vi "ztscopeM Read Waveform Preamble.vi"(0 "Instrument Handle In":i32, 5 "Source":i32(ring) items=["Input Channel 1", "Input Channel 2", "Input Channel 3", "Input Channel 4", "Calc Channel 1", "Calc Channel 2", "Calc Channel 3", "Calc Channel 4", "Ref Channel 1", "Ref Channel 2", "Ref Channel 3", "Ref Channel 4"], 11 "error in":errorcluster) -> (2 "Voltage Offset":dbl, 3 "Voltage Interval":dbl, 4 "Instrument Handle Out":i32, 6 "Type":i32=1, 8 "Points":u32=100, 10 "Acquisition Count":i32=1, 13 "Time Offset":dbl, 14 "Time Interval":dbl=9.99999993922529e-09, 15 "error out":errorcluster)   [LabVIEW 2013]
doc: "Query the selected channel's preamble. The preamble contains all the information necessary to retrieve and interpret a waveform readback."
uses:
  ztscopeM.dll
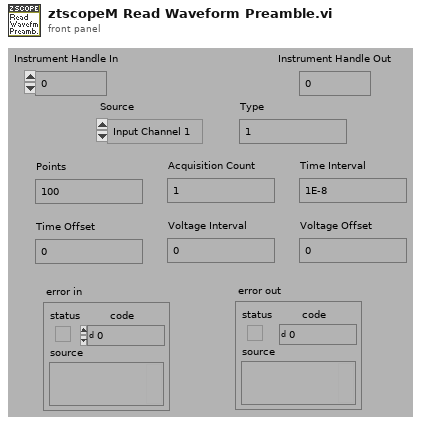
[diagram p1: front panel]
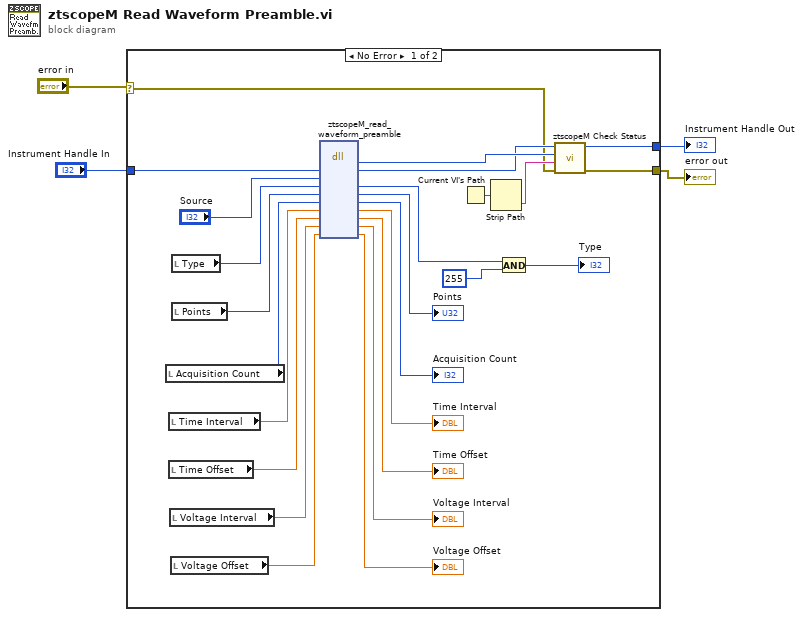
[diagram p0: block diagram]
diagram:
  n1 = case shown="No Error" "error in" {
    selector: "error in" -> [w12 w31]
    tunnel: [w11 w31] -> w1
    tunnel: "Instrument Handle In" -> [w29 w30]
    tunnel: [w10 w30] -> w3
    frame No Error {
      n2 = local read "Acquisition Count"() -> (w24:i32)
      n3 = local read "Time Interval"() -> (w22:dbl)
      n4 = local read "Time Offset"() -> (w20:dbl)
      n5 = local read "Voltage Interval"() -> (w5:dbl)
      n6 = local read "Voltage Offset"() -> (w18:dbl)
      n7 = local read "Type"() -> (w27:i32)
      n8 = local read "Points"() -> (w26:u32)
      n9 = dll-call lib="C:/Program Files/National Instruments/instr.lib/ztscopem/ztscopeM.dll" fn="ztscopeM_read_waveform_preamble"("instrumentHandle"=w29, "source"="Source", "type"=w27, "points"=w26, "acquisitionCount"=w24, "timeInterval"=w22, "timeOffset"=w20, "voltageInterval"=w5, "voltageOffset"=w18) -> (w14:i32, "instrumentHandle"=w13:i32, "type"=w8:i32, "points"=→"Points":u32, "acquisitionCount"=→"Acquisition Count":i32, "timeInterval"=→"Time Interval":dbl, "timeOffset"=→"Time Offset":dbl, "voltageInterval"=→"Voltage Interval":dbl, "voltageOffset"=→"Voltage Offset":dbl)  [unwired: 4 in, 2 out]
      n10 = Current VI's Path() -> (path=w16:path)
      n11 = Strip Path(path=w16) -> (name=w15:string)  [unwired: 1 out]
      n12 = And(x=w8, y=255) -> (x .and. y?=→"Type":i32)
      n13 = call "ztscopeM Check Status.vi"("error in"=w12, "name of VI"=w15, "status"=w14, "instrument handle in"=w13) -> ("error out"=w11:errorcluster, "instrument handle out"=w10:i32)  [unwired: 2 in]
    }
    frame Error {
    }
  }
  "Instrument Handle Out" <- w3
  "error out" <- w1
